vi "1D_Data_to_Igor.vi"(8 "Wave Name":string, 10 "Width":dbl format="%.2f", 11 "Data":dbl[](array[numeric])=[88.25201560693692, 88.167918910518, 88.08981318404682, 88.0168868285138, 87.95089009612809, 87.89039736256106, 87.83704227062073, 87.78920015031018, 87.7485542000132, 87.71337659128233, 87.68541510328214, 87.66287703285205, 87.64756317461499, 87.63764334319724, 87.63495129520638, 87.63764334319724, 87.64756317461499, 87.66287703285205, 87.68541510328214, 87.71337659128233, 87.7485542000132, 87.78920015031018, 87.83704227062073, 87.89039736256106, 87.95089009612809, 88.0168868285138, 88.08981318404682, 88.167918910518, 88.25201560693691] format="%.2f") -> (0 "error out":errorcluster)   [LabVIEW 2014]
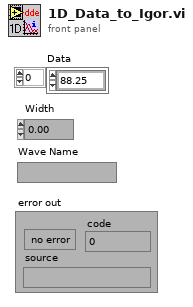
[diagram p1: front panel]
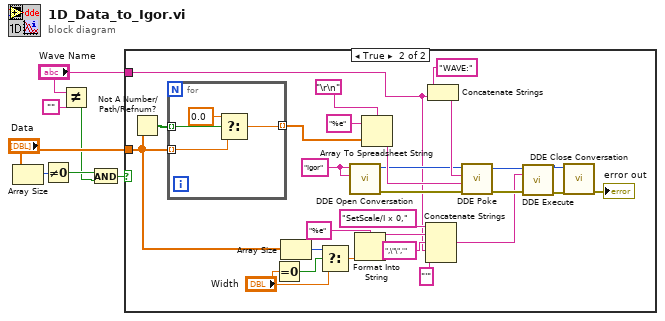
[diagram p0: block diagram]
diagram:
  n1 = Array Size(array="Data") -> (size(s)=w7:i32)
  n2 = Not Equal To 0?(x=w7) -> (x != 0?=w4:bool)
  n3 = Not Equal?(x="Wave Name", y="") -> (x != y?=w1:bool)
  n4 = And(x=w4, y=w1) -> (x .and. y?=w5:bool)
  n5 = case shown="True" w5 {
    tunnel: "Data" -> [_ w11]
    tunnel: "Wave Name" -> [_ w9]
    frame False {
    }
    frame True {
      w34 = "Igor" ("service")
      n6 = Not A Number/Path/Refnum?(number/path/refnum=w11) -> (NaN/Path/Refnum?=w20:bool[])
      n7 = for {
        tunnel: w20 -> [w38] mode=indexing
        tunnel: w11 -> [w37] mode=indexing
        tunnel: [w36] -> w17 mode=indexing
        n8 = Select(t=0.0, s=w38, f=w37) -> (s? t:f=w36:dbl)
      }
      n9 = Equal To 0?(x="Width") -> (x = 0?=w13:bool)
      n10 = Array Size(array=w11) -> (size(s)=w14:i32)
      n11 = Select(t=w14, s=w13, f="Width") -> (s? t:f=w12:dbl)
      n12 = call "DDE Open Conversation.vi"("topic"=w34, "service"=w34) -> ("error out"=w22:errorcluster, "conversation refnum"=w21:u32)  [unwired: 6 in]
      n13 = Format Into String(format string="%e" ("Format String"), w12) -> (resulting string=w30:string)  [unwired: 2 in, 1 out]
      n14 = Array To Spreadsheet String(delimiter (Tab)="\r\n", array=w17, 3:"%e" ("format string")) -> (spreadsheet string=w27:string)
      n15 = Concatenate Strings("SetScale/I x 0," ("Substring"), w30, ",\"\",'" ("Substring"), w9, "'" ("format string")) -> (w23:string)
      n16 = Concatenate Strings("WAVE:", w9) -> (w26:string)
      n17 = call "DDE Poke.vi"("error in (no error)"=w22, "data"=w27, "item"=w26, "conversation refnum in"=w21) -> ("error out"=w24:errorcluster, "conversation refnum out"=w25:u32)  [unwired: 4 in]
      n18 = call "DDE Execute.vi"("error in (no error)"=w24, "command"=w23, "conversation refnum in"=w25) -> ("error out"=w19:errorcluster, "conversation refnum out"=w18:u32)  [unwired: 5 in]
      n19 = call "DDE Close Conversation.vi"("error in (no error)"=w19, "conversation refnum"=w18) -> ("error out"=→"error out":errorcluster)  [unwired: 7 in]
    }
  }
